vi "oax_Save Extracted.vi"(0 "File Path (.wav)":path=path "C:/Program Files/National Instruments/LabVIEW 8.2/examples/Order Analysis/Demo VI/Example Data/DownAcc.wav", 1 "OK?":bool, 5 "orders to extract out":dbl[](array[numeric]), 7 "Vibration signals":waveform(dbl)[](array[waveform]), 9 "speed profile":T3 {"speed [RPM]" format="%.2f"; "time [s]" format="%.2f"}, 11 "error in":errorcluster, 12 "window info":T1={"window type"=62, "window length"=2048} {"window type" items=["None"=0, "Hanning"=1, "Hamming"=2, "Blackman-Harris"=3, "Exact Blackman"=4, "Blackman"=5, "Flat Top"=6, "4 Term B-Harris"=7, "7 Term B-Harris"=8, "Low Sidelobe"=9, "Gaussian"=62]; "window length" min=0}, 13 "bandwidth":T2={"bandwidth"=1.0, "unit"=enum."Order"}, 14 "Fs":dbl) -> (15 "error out":errorcluster)   [LabVIEW 2017]
uses:
  <vilib>/addons/Sound and Vibration/Order Analysis/Tach Process/SubVIs/speed profile.ctl
  <vilib>/addons/Sound and Vibration/Order Analysis/Ref Gabor Order Tracking/window information.ctl
  <vilib>/sound2/lvsound2.llb/Sound Data Format.ctl
  <vilib>/sound2/lvsound2.llb/Sound File Write (DBL).vi
  <vilib>/sound2/lvsound2.llb/Sound File Write Open.vi
  <vilib>/addons/Sound and Vibration/Order Analysis/Gabor Order Tracking/OAT Extract Order Waveforms (Combined Orders).vi
  <vilib>/addons/Sound and Vibration/Order Analysis/Gabor Order Tracking/SoundVib_Gabor.lvlib
  <vilib>/addons/Sound and Vibration/Order Analysis/Tach Process/SoundVib_TachProcess.lvlib
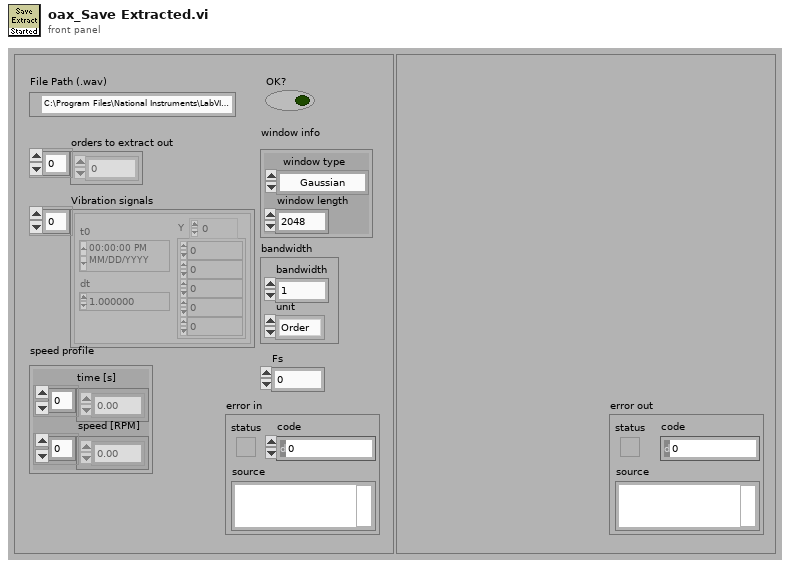
[diagram p1: front panel]
types:
  T1 = typedef "SoundVib_Gabor.lvlib/window information.ctl" = cluster{"window type":u32, "window length":i32}
  T2 = cluster{"bandwidth":dbl, "unit":enum16{"Order", "Hz"}}
  T3 = typedef "SoundVib_TachProcess.lvlib/speed profile.ctl" = cluster{"time [s]":dbl[], "speed [RPM]":dbl[]}
  T4 = typedef "Sound Data Format.ctl" = cluster{"sample rate (S/s)":dbl, "number of channels":i32, "bits per sample":i32}
  T5 = enum16{"open", "replace", "create", "open or create", "replace or create", "replace or create with confirmation"}
  T6 = typedef "Sound File Refnum.ctl" = refnum<file>
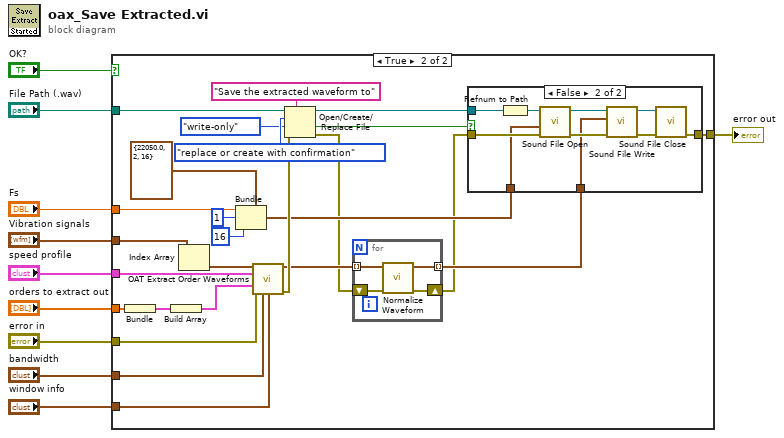
[diagram p0: block diagram]
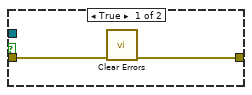
[diagram p3: hidden frame]
diagram:
  n1 = case shown="True" "OK?" {
    tunnel: "error in" -> [w11 w35]
    tunnel: [w11 w25] -> w1
    tunnel: "Fs" -> [_ w37]
    tunnel: "Vibration signals" -> [_ w33]
    tunnel: "File Path (.wav)" -> [_ w22]
    tunnel: "orders to extract out" -> [_ w32]
    tunnel: "speed profile" -> [_ w30]
    tunnel: "bandwidth" -> [_ w29]
    tunnel: "window info" -> [_ w28]
    frame False {
    }
    frame True {
      n2 = Bundle("orders to extract out"=w32) -> (w36:cluster{"orders to extract out":dbl[]})  [unwired: 1 in]
      n3 = Build Array(w36) -> (w31:cluster{"orders to extract out":dbl[]}[])
      n4 = Index Array(array=w33) -> (element=w34:waveform(dbl))  [unwired: 1 in]
      n5 = Bundle(cluster=T4 {"sample rate (S/s)"=22050.0, "number of channels"=2, "bits per sample"=16} ("sound format"), "sample rate (S/s)"=w37, "number of channels"=1, "bits per sample"=16) -> (w17:T4)
      n6 = call-poly <vilib>:"OAT Extract Order Waveforms.vi"("scaled signal [EU]"=w34, "speed profile"=w30, "orders to extract"=w31, "error in (no error)"=w35, "bandwidth"=w29, "window info"=w28) -> ("order waveforms"=w15:waveform(dbl)[], "error out"=w18:errorcluster)  [unwired: 5 in, 3 out]
      n7 = Open/Create/Replace File(file path (use dialog)=w22, error in=w18, prompt="Save the extracted waveform to", operation (0:open)=T5."replace or create with confirmation", access (0:read/write)=enum16{"read/write", "read-only", "write-only"}."write-only") -> (refnum out=w20:refnum<file>, cancelled=w19:bool, error out=w13:errorcluster)  [unwired: 1 in]
      n8 = for {
        tunnel: w15 -> [w41] mode=indexing
        tunnel: [w40] -> w14 mode=indexing
        shift-right: [w38] -> w12
        shift-left: w13 -> [w39]
        n9 = call <vilib>:"Normalize Waveform.vi"("error in (no error)"=w39, "waveform in"=w41) -> ("error out"=w38:errorcluster, "normalized waveform"=w40:waveform(dbl))  [unwired: 6 in, 2 out]
      }
      n10 = case shown="False" w19 {
        tunnel: w12 -> [w43 w51]
        tunnel: [w42 w48] -> w25
        tunnel: w14 -> [_ w44]
        tunnel: w20 -> [_ w47]
        tunnel: w17 -> [_ w45]
        frame True {
          n11 = call <vilib>:"Clear Errors.vi"("error in (no error)"=w43) -> ("error out"=w42:errorcluster)  [unwired: 5 in, 1 out]
        }
        frame False {
          n12 = Refnum to Path(1:w47) -> (0:w46:path)
          n13 = call-poly <vilib>:"Sound File Open.vi"("error in (no error)"=w51, "sound format"=w45, "path"=w46) -> ("error out"=w52:errorcluster, "sound file refnum"=w53:T6)  [unwired: 7 in]
          n14 = call-poly <vilib>:"Sound File Write.vi"("error in (no error)"=w52, "data"=w44, "sound file refnum"=w53) -> ("error out"=w50:errorcluster, "sound file refnum out"=w49:T6)  [unwired: 7 in]
          n15 = call <vilib>:"Sound File Close.vi"("error in (no error)"=w50, "sound file refnum"=w49) -> ("error out"=w48:errorcluster)  [unwired: 9 in]
        }
      }
    }
  }
  "error out" <- w1
